vi "NF87xx.evt call Absolute Move.vi"(0 "i ref in":refnum<vi>, 1 "Instance":string="N/A", 2 "forward?":bool, 4 "velocity (10 .. 2000)":dbl=10.0 min=10.0 max=2000.0, 5 "error in (no error)":errorcluster, 6 "System":string="N/A") -> (14 "i ref out":refnum<vi>, 19 "error out":errorcluster)   [LabVIEW 2014, in "NF87XX.lvlib"]
doc: "This VI sets the \"AbsMove\" case by a notification call. The instance has to be something else but N/A."
uses:
  NF87XX.lvlib
  CS_Core/CSSystem/CoreLib/CoreLib.double 2 byte array.vi
  CS_Core/CSSystem/CoreLib/CoreLib.short 2 byte array.vi
  CS_Core/CSSystem/CoreLib/CoreLib.string 2 byte array.vi
  CS_Core/BaseProcess/BaseProcess.lvlib
  CS_Core/CSSystem/CoreLib/CoreLib.lvlib
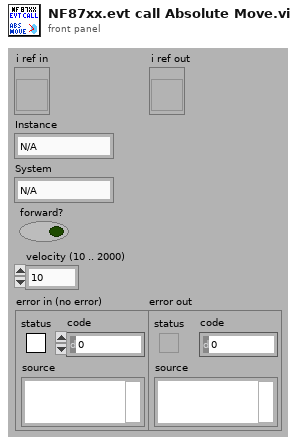
[diagram p1: front panel]
types:
  T1 = enum16{"simple", "synchronous", "asynchronous", "notification"}
  T2 = typedef "CoreDefs.rawDataType.ctl" = i8[]
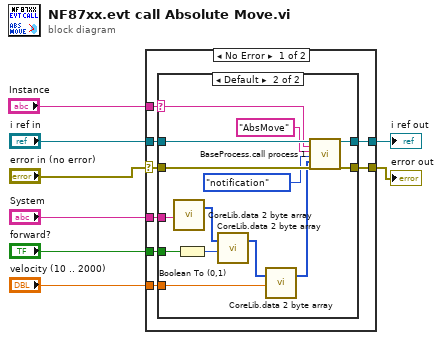
[diagram p0: block diagram]
diagram:
  n1 = case shown="No Error" "error in (no error)" {
    selector: "error in (no error)" -> [w10 w33]
    tunnel: [w16 w34] -> w8
    tunnel: [w15 w33] -> w7
    tunnel: "i ref in" -> [w14 w34]
    tunnel: "forward?" -> [w13 _]
    tunnel: "velocity (10 .. 2000)" -> [w12 _]
    tunnel: "Instance" -> [w11 _]
    tunnel: "System" -> [w9 _]
    frame No Error {
      n2 = case shown="Default" w11 {
        selector: w11 -> [_ w27]
        tunnel: [w18 w32] -> w16
        tunnel: [w17 w31] -> w15
        tunnel: w14 -> [w18 w30]
        tunnel: w10 -> [w17 w29]
        tunnel: w13 -> [_ w26]
        tunnel: w12 -> [_ w28]
        tunnel: w9 -> [_ w25]
        frame "N/A" {
        }
        frame Default {
          n3 = call-poly "CoreLib.data 2 byte array.vi"("string"=w25) -> ("byteArray out"=w21:T2)  [unwired: 18 in]
          n4 = Boolean To (0,1)(Boolean=w26) -> (0, 1=w20:i16)
          n5 = call-poly "CoreLib.data 2 byte array.vi"("byteArray"=w21, "i16"=w20) -> ("byteArray out"=w19:T2)  [unwired: 17 in]
          n6 = call-poly "CoreLib.data 2 byte array.vi"("byteArray"=w19, "f64"=w28) -> ("byteArray out"=w22:T2)  [unwired: 17 in]
          n7 = call "BaseProcess.call process 1.vi"("i ref in"=w30, "Object"=w27, "Selector"="AbsMove", "CallType"=T1."notification", "Data"=w22, "error in (no error)"=w29) -> ("i ref out"=w32:refnum<vi>, "error out"=w31:errorcluster)  [unwired: 11 in, 1 out]
        }
      }
    }
    frame Error {
    }
  }
  "error out" <- w7
  "i ref out" <- w8
